vi "Sub_FFT.vi"(2 "Start/End":cluster{"START":dbl, "END":dbl}[](array[cluster]) {"END" min=0.0 max=1000.0 step=1.0 format="%#.0f"; "START" min=0.0 max=1000.0 step=1.0 format="%#.0f"}, 3 "HBN":dbl[](array[numeric])) -> (0 "Ok 2":bool, 1 "Start/End 2":cluster{"START":dbl, "END":dbl}[](array[cluster]) {"END" min=0.0 max=1000.0 step=1.0 format="%#.1g"; "START" min=0.0 max=1000.0 step=1.0 format="%#.1g"})   [LabVIEW 2020]
uses:
  <vilib>/Analysis/NI_AAL_SigProc.lvlib
panel:
  in  "Y Scale":dbl(slide) min=0.0 step=1.0 scale=10.0..0.01
  out "Graph_FFT":cluster{"rms_sign":dbl[]}[](graph)
  in  "ENTRY":i8 min=0 max=100 step=1
  in  "Ok":bool
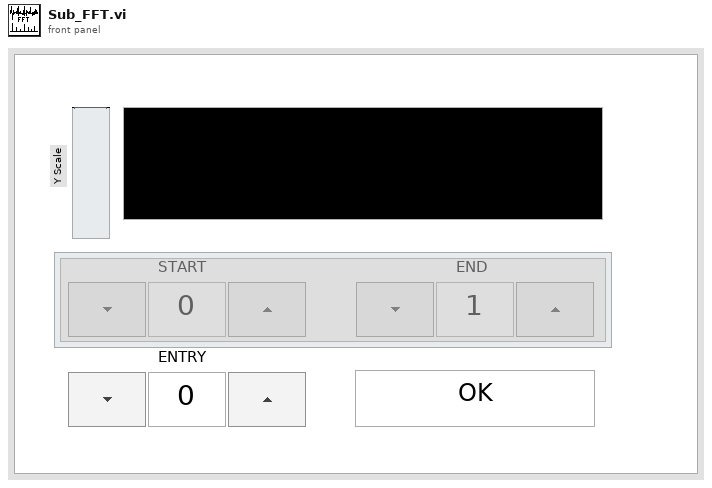
[diagram p1: front panel]
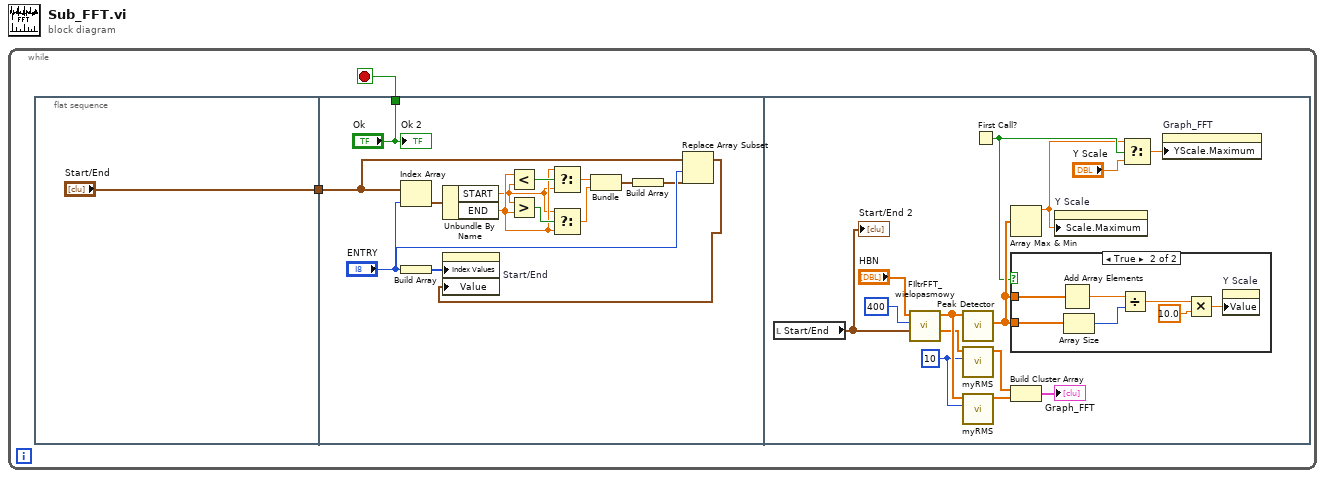
[diagram p0: block diagram]
diagram:
  n1 = while {
    stop <- w2 stop-if-true
    n2 = flat-sequence {
      tunnel: ["Start/End"] -> w1
      tunnel: ["Ok"] -> w2
      tunnel: w1 -> [w4]
      frame #0 {
      }
      frame #1 {
        n3 = Index Array(array=w4, index="ENTRY") -> (element=w8:cluster{"START":dbl, "END":dbl})
        n4 = Build Array("ENTRY") -> (w16:i8[])
        n5 = Unbundle By Name(w8) -> ("START"=w10:dbl, "END"=w11:dbl)
        n6 = Less?(x=w11, y=w10) -> (x < y?=w14:bool)
        n7 = Greater?(x=w10, y=w11) -> (0:w15:bool)
        n8 = Select(t=w11, s=w14, f=w10) -> (s? t:f=w12:dbl)
        n9 = Select(t=w10, s=w15, f=w11) -> (s? t:f=w13:dbl)
        n10 = Bundle("START"=w12, "END"=w13) -> (w9:cluster{"START":dbl, "END":dbl})  [unwired: 1 in]
        n11 = Build Array(w9) -> (w6:cluster{"START":dbl, "END":dbl}[])
        n12 = Replace Array Subset(array=w4, new element=w6, index="ENTRY") -> (w5:cluster{"START":dbl, "END":dbl}[])
        n13 = property on="Start/End" class="Arr (strict)"("Index Values"=w16, "Value"=w5) -> ()  [unwired: 2 in, 2 out]
        "Ok 2" <- "Ok"
      }
      frame #2 {
        w20 = 10 ("LptRMS")
        n14 = local read "Start/End"() -> (w18:cluster{"START":dbl, "END":dbl}[])
        "Start/End 2" <- w18
        n15 = call "FIltrFFT_wielopasmowy.vi"("zakresy"=w18, "f_sampl [kHz]"=400, "dane"="HBN") -> ("FFTcut"=w22:cdb[], "FFT"=w26:cdb[])  [unwired: 5 in, 2 out]
        n16 = call <vilib>:"Peak Detector.vi"("X"=w26) -> ("Amplitudes"=w31:dbl[])  [unwired: 6 in, 4 out]
        n17 = call "myRMS.vi"("LptRMS"=w20, "dane"=w22) -> ("rms_sign"=w24:dbl[])  [unwired: 9 in]
        n18 = call "myRMS.vi"("LptRMS"=w20, "dane"=w26) -> ("rms_sign"=w25:dbl[])  [unwired: 9 in]
        n19 = First Call?() -> (First Call?: T/F=w29:bool)
        n20 = Array Max & Min(array=w31) -> (max value=w28:dbl)  [unwired: 3 out]
        n21 = case shown="True" w29 {
          tunnel: w31 -> [_ w36]
          tunnel: w31 -> [_ w35]
          frame False {
          }
          frame True {
            n22 = Add Array Elements(numeric array=w35) -> (sum=w37:dbl)
            n23 = Array Size(array=w36) -> (size(s)=w38:i32)
            n24 = Divide(x=w37, y=w38) -> (x/y=w34:dbl)
            n25 = Multiply(x=w34, y=10.0) -> (x*y=w32:dbl)
            n26 = property on="Y Scale" class="Slide (strict)"("Value"=w32) -> ()  [unwired: 2 in, 2 out]
          }
        }
        n27 = Build Cluster Array(w24, w25) -> (→"Graph_FFT":cluster{"rms_sign":dbl[]}[])
        n28 = property on="Y Scale" class="Slide (strict)"("Scale.Maximum"=w28) -> ()  [unwired: 2 in, 2 out]
        n29 = Select(t=w28, s=w29, f="Y Scale") -> (s? t:f=w30:dbl)
        n30 = property on="Graph_FFT" class="WFGraph (strict)"("YScale.Maximum"=w30) -> ()  [unwired: 2 in, 2 out]
      }
    }
  }
